vi "Execute.vi"(6 "Index [-1]":i32=-1, 7 "Composite Object":refnum<class "CConfig Object.lvclass">, 8 "error in (no error)":errorcluster, 9 "Results":string[][](array[string]), 11 "Config Query in":refnum<class "Insert Query.lvclass">) -> (0 "error out":errorcluster, 1 "Results":string[][](array[string]), 2 "Result":bool, 3 "Config Query out":refnum<class "Insert Query.lvclass">, 4 "Index":i32, 5 "Composite Object":refnum<class "CConfig Object.lvclass">)   [LabVIEW 2013, in "Insert Query.lvclass"]
doc: "Copyright 2018, Carya Automatisering, Wiebe Walstra."
uses:
  Insert Query.lvclass
  CConfig Object.lvclass
  Insert Query.lvclass/Insert Query.ctl
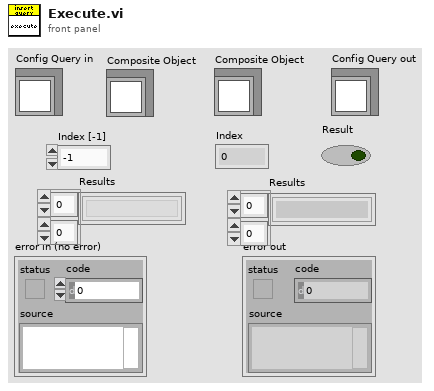
[diagram p1: front panel]
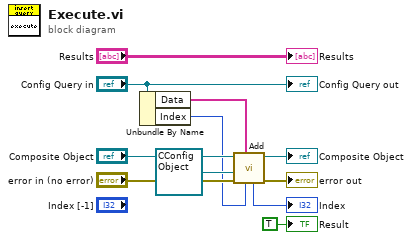
[diagram p0: block diagram]
diagram:
  n1 = Unbundle By Name("Config Query in") -> ("Data"=w2:string[], "Index"=w1:i32)
  n2 = call-dynamic "Add.vi"("Index [-1, last]"=w1, "Data"=w2, "error in (no error)"="error in (no error)", "Child"=refnum<class "CConfig Object.lvclass"> refnum, "Composite Object in"="Composite Object") -> ("error out"=→"error out":errorcluster, "Composite Object out"=→"Composite Object":refnum<class "CConfig Object.lvclass">, "Index"=→"Index":i32)  [unwired: 4 in]
  "Config Query out" <- "Config Query in"
  "Result" <- TRUE ("Result")
  "Results" <- "Results"
